vi "Square Root Keep Sign.vi"(1 "Input":dbl) -> (0 "Square Root Save Sign":dbl)   [LabVIEW 2018]
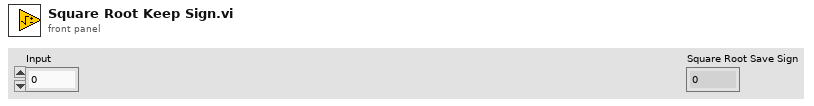
[diagram p1: front panel]
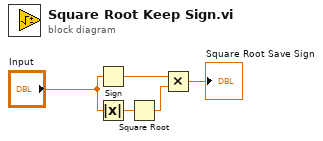
[diagram p0: block diagram]
diagram:
  n1 = Sign(1:"Input") -> (0:w3:dbl)
  n2 = Absolute Value(x="Input") -> (abs(x)=w5:dbl)
  n3 = Square Root(x=w5) -> (sqrt(x)=w4:dbl)
  n4 = Multiply(x=w3, y=w4) -> (x*y=→"Square Root Save Sign":dbl)
